vi "PDE_Find First Error.vi"(10 "PDE Error":T1[](array[typedef]), 11 "Failure":bool[](array[boolean])) -> (3 "first error":T1)   [LabVIEW 2017, in "NI_PDE.lvlib"]
uses:
  <vilib>/gmath/NI_PDE.lvlib
  <vilib>/gmath/pde.llb/Common/PDE_Error.ctl
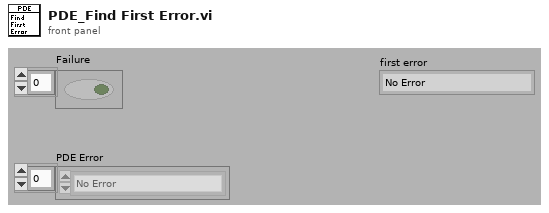
[diagram p1: front panel]
types:
  T1 = typedef "NI_PDE.lvlib/PDE_Error.ctl" = enum16{"No Error", "k is zero", "End point <= start point", "# of time steps < 2", "# of spatial points < 3", "# of grid < 1 for FEM", "# of boundary < 3 for FEM", "Incompatible RHS size", "Incompatible BC size", "Incompatible IC size", "PDE class conflict", "RHS class conflict", "Domain class conflict", "BC class conflict", "IC class conflict"}
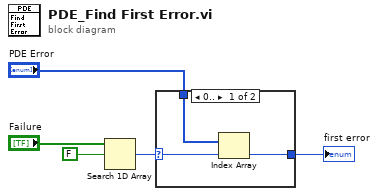
[diagram p0: block diagram]
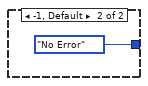
[diagram p2: hidden frame]
diagram:
  n1 = Search 1D Array(1D array="Failure", element=FALSE) -> (index of element=w4:i32)  [unwired: 1 out]
  n2 = case shown="0.." w4 {
    selector: w4 -> [w8 _]
    tunnel: [w7 PDE_Error."No Error" ("Error")] -> w2
    tunnel: "PDE Error" -> [w6 _]
    frame 0.. {
      n3 = Index Array(array=w6, index=w8) -> (element=w7:T1)
    }
    frame -1, Default {
    }
  }
  "first error" <- w2
